vi "Transport Problem to Linear Programming.vi"(3 "Transport Costs":dbl[][](array[numeric]) min=0.0 format="%.2f", 4 "Traders":cluster{"name":string, "produced units":dbl}[](array[cluster]) {"produced units" format="%.2f"}, 5 "Producers":cluster{"name":string, "produced units":dbl}[](array[cluster]) {"produced units" format="%.2f"}) -> (0 "error":i32, 1 "Solution":dbl[][](array[numeric]) format="%.2f", 2 "minimal cost":dbl format="%.2f")   [LabVIEW 2017, in "NI_Gmath.lvlib"]
uses:
  <vilib>/gmath/NI_Gmath.lvlib
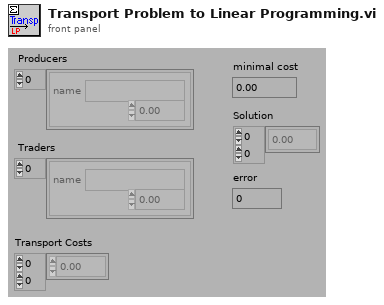
[diagram p1: front panel]
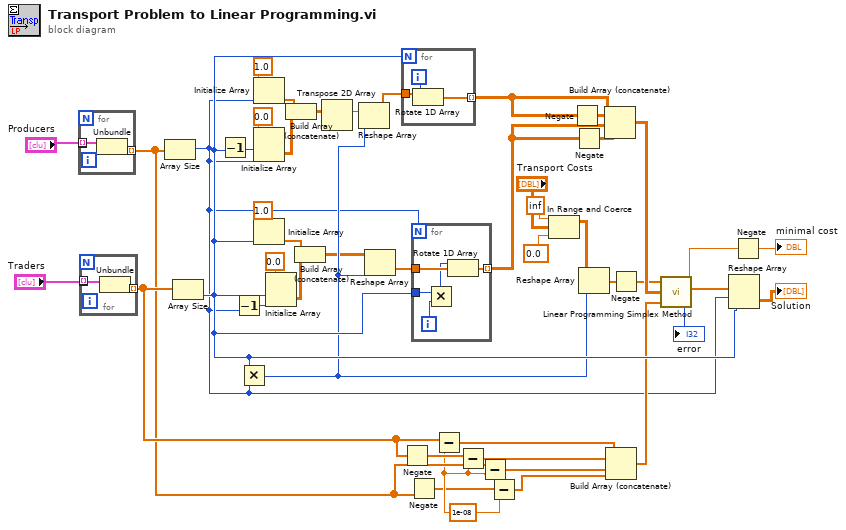
[diagram p0: block diagram]
diagram:
  w8 = 1e-08
  n1 = for {
    tunnel: [w48] -> _ mode=indexing
    tunnel: "Producers" -> [w48] mode=indexing
    tunnel: [w47] -> w9 mode=indexing
    n2 = Unbundle(w48) -> ("produced units"=w47:dbl)  [unwired: 1 out]
  }
  n3 = for {
    tunnel: "Traders" -> [w50] mode=indexing
    tunnel: [w50] -> _ mode=indexing
    tunnel: [w49] -> w13 mode=indexing
    n4 = Unbundle(w50) -> ("produced units"=w49:dbl)  [unwired: 1 out]
  }
  n5 = Array Size(array=w9) -> (size(s)=w15:i32)
  n6 = Array Size(array=w13) -> (size(s)=w45:i32)
  n7 = Decrement(x=w45) -> (x-1=w31:i32)
  n8 = Decrement(x=w15) -> (x-1=w23:i32)
  n9 = Multiply(x=w45, y=w15) -> (x*y=w44:i32)
  n10 = Initialize Array(1.0, w15) -> (w37:dbl[])
  n11 = Initialize Array(0.0, w31, w15) -> (w29:dbl[][])
  n12 = Initialize Array(1.0, w45) -> (w24:dbl[])
  n13 = Initialize Array(0.0, w45, w23) -> (w25:dbl[][])
  n14 = Build Array (concatenate)(w37, w29) -> (w30:dbl[][])
  n15 = Build Array (concatenate)(w24, w25) -> (w26:dbl[][])
  n16 = Transpose 2D Array(2D array=w30) -> (transposed array=w32:dbl[][])
  n17 = Reshape Array(w32, w44) -> (w28:dbl[])
  n18 = Reshape Array(w26, w44) -> (w27:dbl[])
  n19 = for {
    N: w45 -> [_]
    tunnel: w28 -> [w53]
    tunnel: [w52] -> w33 mode=indexing
    i -> [w51]
    n20 = Rotate 1D Array(1:w53, 2:w51) -> (0:w52:dbl[])
  }
  n21 = Negate(x=w13) -> (-x=w12:dbl[])
  n22 = Negate(x=w9) -> (-x=w7:dbl[])
  n23 = for {
    N: w15 -> [_]
    tunnel: w27 -> [w58]
    tunnel: w45 -> [w57]
    tunnel: [w56] -> w35 mode=indexing
    i -> [w55]
    n24 = Multiply(x=w57, y=w55) -> (x*y=w54:i32)
    n25 = Rotate 1D Array(1:w58, 2:w54) -> (0:w56:dbl[])
  }
  n26 = Subtract(x=w13, y=w8) -> (x-y=w11:dbl[])
  n27 = Subtract(x=w12, y=w8) -> (x-y=w10:dbl[])
  n28 = Subtract(x=w9, y=w8) -> (x-y=w6:dbl[])
  n29 = Subtract(x=w7, y=w8) -> (x-y=w5:dbl[])
  n30 = In Range and Coerce(upper limit=inf, x="Transport Costs", lower limit=0.0) -> (coerced(x)=w1:dbl[][])  [unwired: 1 out]
  n31 = Negate(x=w33) -> (-x=w34:dbl[][])
  n32 = Negate(x=w35) -> (-x=w36:dbl[][])
  n33 = Reshape Array(w1, w44) -> (w39:dbl[])
  n34 = Build Array (concatenate)(w33, w34, w35, w36) -> (w42:dbl[][])
  n35 = Build Array (concatenate)(w11, w10, w6, w5) -> (w38:dbl[])
  n36 = Negate(x=w39) -> (-x=w40:dbl[])
  n37 = call <vilib>:"Linear Programming Simplex Method.vi"("C"=w40, "M"=w42, "B"=w38) -> ("maximum"=w41:dbl, "X"=w43:dbl[], "error"=→"error":i32)  [unwired: 1 out]
  n38 = Reshape Array(w43, w15, w45) -> (→"Solution":dbl[][])
  n39 = Negate(x=w41) -> (-x=→"minimal cost":dbl)
